vi "fold onto itself.vi"(9 "whatever":dbl[](array[numeric]), 10 "omega":dbl[](array[numeric]), 11 "window size":dbl=1.0) -> (1 "whatever out":dbl[](array[numeric]), 2 "omega out":dbl[](array[numeric]))   [LabVIEW 2010]
panel:
  out "x+y":dbl[](array[numeric])
  out "Numeric":dbl
  out "x*y":dbl
  out "x+1":i32
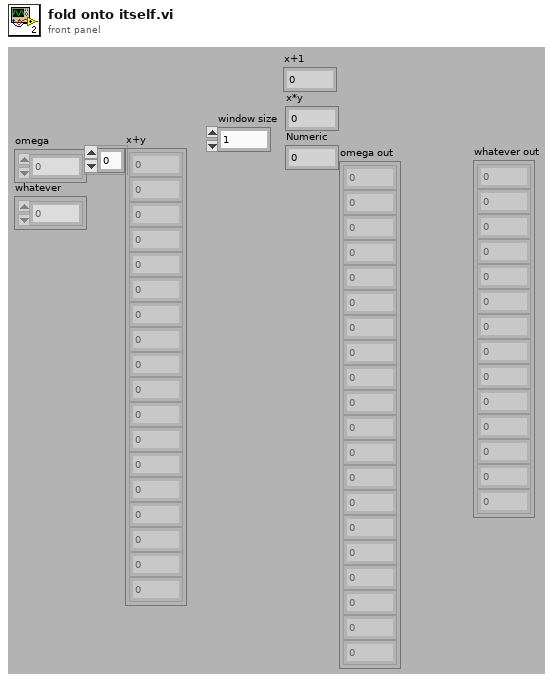
[diagram p1: front panel]
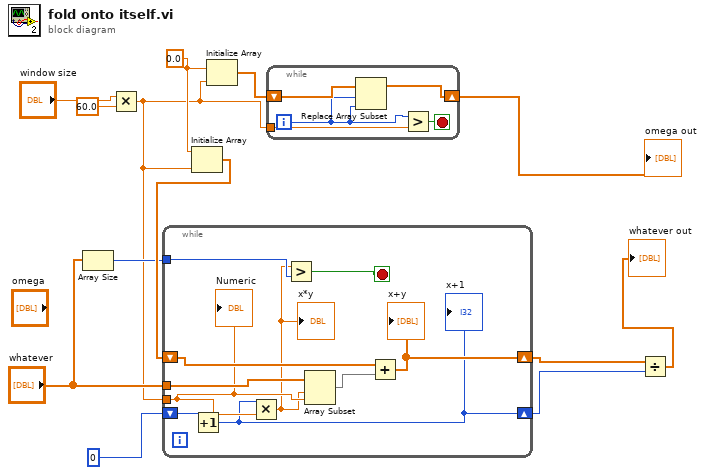
[diagram p0: block diagram]
diagram:
  w9 = 0.0 ("element")
  n1 = Array Size(array="whatever") -> (size(s)=w2:i32)
  n2 = Multiply(x="window size", y=60.0) -> (x*y=w1:dbl)
  n3 = Initialize Array(w9, w1) -> (w8:dbl[])
  n4 = while {
    shift-right: [w15] -> w6
    shift-left: w8 -> [w22]
    tunnel: "whatever" -> [w23]
    tunnel: w1 -> [w21]
    shift-right: [w14] -> w5
    shift-left: 0 ("element") -> [w20]
    tunnel: w2 -> [w19]
    stop <- w17 stop-if-true
    n5 = Increment(x=w20) -> (x+1=w14:i32)
    "x+1" <- w14
    n6 = Multiply(x=w14, y=w21) -> (x*y=w18:dbl)
    "x*y" <- w18
    n7 = Greater?(x=w18, y=w19) -> (0:w17:bool)
    n8 = Array Subset(array=w23, index=w18, length=w21) -> (w16:dbl[])
    n9 = Add(x=w22, y=w16) -> (x+y=w15:dbl[])
    "x+y" <- w15
    "Numeric" <- w21
  }
  n10 = Initialize Array(w9, w1) -> (w11:dbl[])
  n11 = while {
    shift-right: [w27] -> w10
    shift-left: w11 -> [w28]
    tunnel: w1 -> [w24]
    i -> [w25]
    stop <- w26 stop-if-true
    n12 = Replace Array Subset(array=w28, new element=w25, index=w25) -> (w27:dbl[])
    n13 = Greater?(x=w25, y=w24) -> (0:w26:bool)
  }
  "omega out" <- w10
  n14 = Divide(x=w6, y=w5) -> (x/y=→"whatever out":dbl[])
